vi "RSZVB Start Calibration Line.vi"(6 "Port 2 (1)":i32=1, 7 "Port 1 (1)":i32=1, 8 "error in (no error)":errorcluster {"code" format="%.0x"}, 9 "Line (1)":i32=1, 10 "Channel (1)":i32=1, 11 "VISA session":refnum<visa-resource-name>) -> (0 "error out":errorcluster {"code" format="%.0x"}, 3 "dup VISA session":refnum<visa-resource-name>)   [LabVIEW 2011]
doc: "This VI starts a calibration measurement in order to acquire measurement data for the selected line.\n\nRemote-control command(s):\n[SENSe<Ch>:]CORRection:COLLect[:ACQuire]:SELected LINEN,<line> <port_no>[,<port_no>]"
uses:
  _utility/RSZVB Global Data.vi
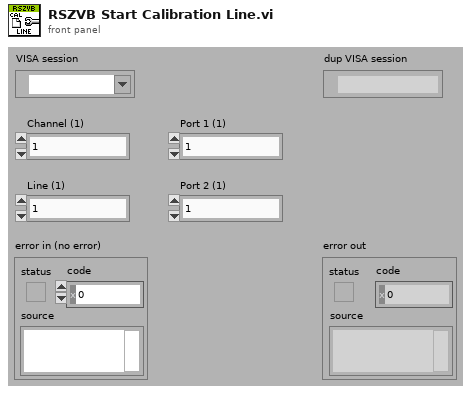
[diagram p1: front panel]
types:
  T1 = cluster{"Error Checking (T: On)":bool, "Installed Options":string[], "Data Valid?":bool, "Ports":i32, "Model":string[], "Option Checking (T: On)":bool}[]
  T2 = cluster{"Error Checking (T: On)":bool, "Installed Options":string[], "Data Valid?":bool, "Ports":i32, "Model":string[], "Option Checking (T: On)":bool}
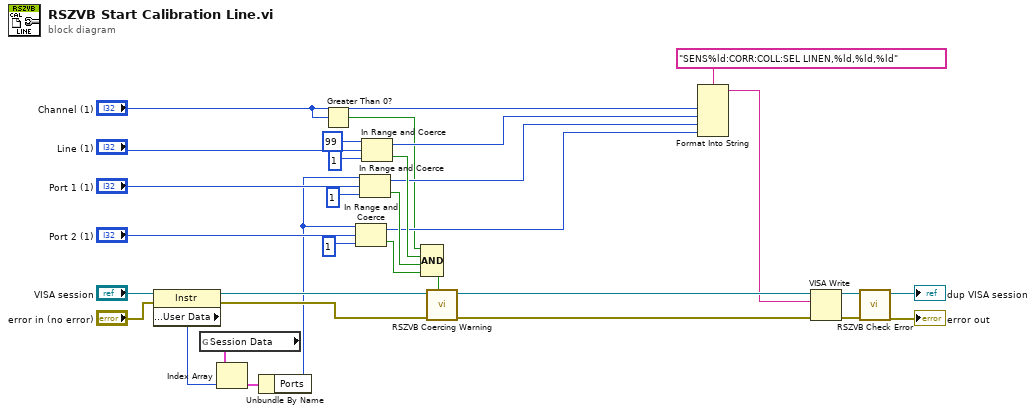
[diagram p0: block diagram]
diagram:
  n1 = property class="Instr"(reference="VISA session", error in="error in (no error)") -> (reference out=w23:refnum<visa-resource-name>, error out=w24:errorcluster, "General Settings:User Data"=w25:u32)
  n2 = global read "RSZVB Global Data.vi" "Session Data"() -> (w26:T1)
  n3 = Index Array(array=w26, index=w25) -> (element=w27:T2)
  n4 = Unbundle By Name(w27) -> ("Ports"=w1:i32)
  n5 = Greater Than 0?(x="Channel (1)") -> (x > 0?=w3:bool)
  n6 = In Range and Coerce(upper limit=w1, x="Port 2 (1)", lower limit=1) -> (coerced(x)=w4:i32, In Range?=w8:bool)
  n7 = In Range and Coerce(upper limit=w1, x="Port 1 (1)", lower limit=1) -> (coerced(x)=w5:i32, In Range?=w29:bool)
  n8 = In Range and Coerce(upper limit=99 ("lower limit"), x="Line (1)", lower limit=1) -> (coerced(x)=w6:i32, In Range?=w7:bool)
  n9 = Compound Arithmetic op=AND(w3, w7, w29, w8) -> (w28:bool)
  n10 = call "RSZVB Coercing Warning.vi"("In Range?"=w28, "error in (no error)"=w24, "VISA session"=w23) -> ("error out"=w13:errorcluster, "dup VISA session"=w14:refnum<visa-resource-name>)  [unwired: 7 in]
  n11 = Format Into String(format string="SENS%ld:CORR:COLL:SEL LINEN,%ld,%ld,%ld", "Channel (1)", w6, w5, w4) -> (resulting string=w10:string)  [unwired: 2 in, 1 out]
  n12 = VISA Write(VISA resource name=w14, write buffer=w10, error in (no error)=w13) -> (VISA resource name out=w30:refnum<visa-resource-name>, error out=w31:errorcluster)  [unwired: 1 out]
  n13 = call "RSZVB Check Error.vi"("error in (no error)"=w31, "VISA session"=w30) -> ("error out"=→"error out":errorcluster, "dup VISA session"=→"dup VISA session":refnum<visa-resource-name>)  [unwired: 8 in]
